vi "Get Current DateTime.vi"(9 "Leading Apostrophe":bool) -> (0 "Current Timestamp":timestamp, 1 "Time String":string, 2 "Date String":string, 3 "Date/Time String":string)   [LabVIEW 2021]
panel:
  # "Used to Trick Excel \ninto accepting\nString as Text\ninstead of Number"
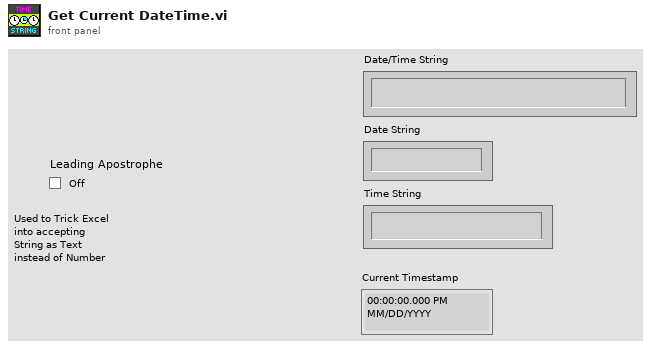
[diagram p1: front panel]
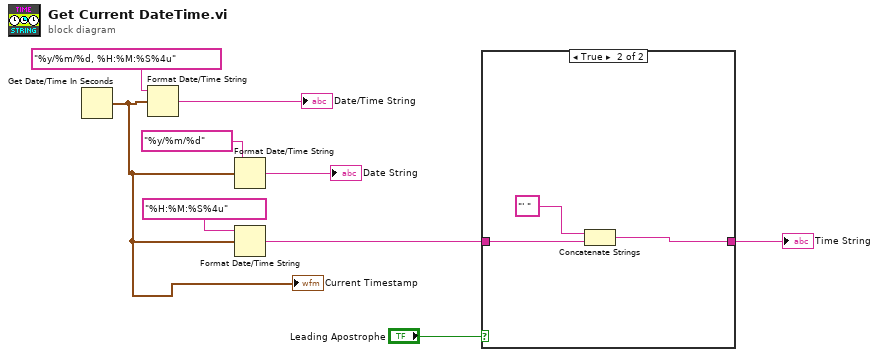
[diagram p0: block diagram]
diagram:
  n1 = Get Date/Time In Seconds() -> (seconds since 1Jan1904=w4:timestamp)
  "Current Timestamp" <- w4
  n2 = Format Date/Time String(time format string (%c)="%y/%m/%d, %H:%M:%S%4u", seconds (now)=w4) -> (date/time string=→"Date/Time String":string)  [unwired: 1 in]
  n3 = Format Date/Time String(time format string (%c)="%y/%m/%d", seconds (now)=w4) -> (date/time string=→"Date String":string)  [unwired: 1 in]
  n4 = Format Date/Time String(time format string (%c)="%H:%M:%S%4u", seconds (now)=w4) -> (date/time string=w2:string)  [unwired: 1 in]
  n5 = case shown="True" "Leading Apostrophe" {
    tunnel: w2 -> [w10 w12]
    tunnel: [w10 w11] -> w1
    frame False {
    }
    frame True {
      n6 = Concatenate Strings("' " ("string"), w12) -> (w11:string)
    }
  }
  "Time String" <- w1
